vi "Index not Created Invalid path.vi"(8 "error in (no error)":errorcluster, 11 "Indexing Test Finder Test in":refnum<class "Indexing Test Finder Test.lvclass">) -> (0 "error out":errorcluster, 3 "Indexing Test Finder Test out":refnum<class "Indexing Test Finder Test.lvclass">)   [LabVIEW 2020, in "LUnit Tests.lvlib" / "Indexing Test Finder Test.lvclass"]
uses:
  Indexing Test Finder Test.lvclass
  Indexing Test Finder Test.lvclass/Indexing Test Finder Test.ctl
  source/Framework/Helper Classes/Test Finder/Test Finder.lvclass
  Test Finder/Finder Test.lvclass
  c59a45e6-8387-4d73-9fe8-839093b27eb6.vi
  <vilib>/Astemes/LUnit/Test Case.lvclass
  C:/Git/astemes-lunit/tests/Test Finder/Finder Test.lvclass
  C:/Program Files (x86)/National Instruments/LabVIEW 2020/vi.lib/Astemes/LUnit/Test Case.lvclass
  C:/Git/astemes-lunit/tests/Indexing Test Finder Test/Indexing Test Finder Test.lvclass
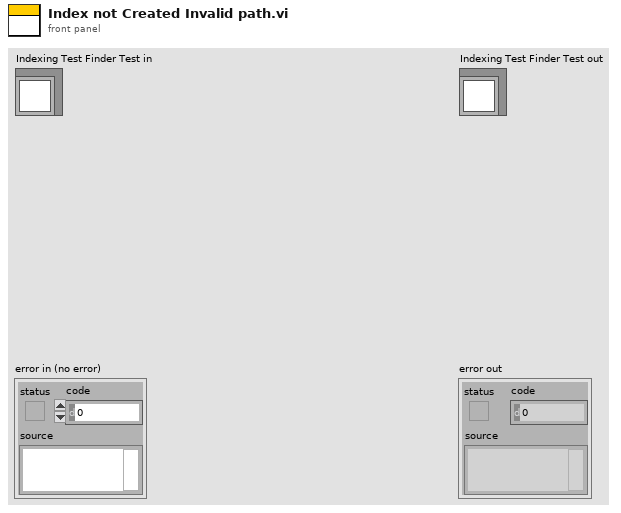
[diagram p1: front panel]
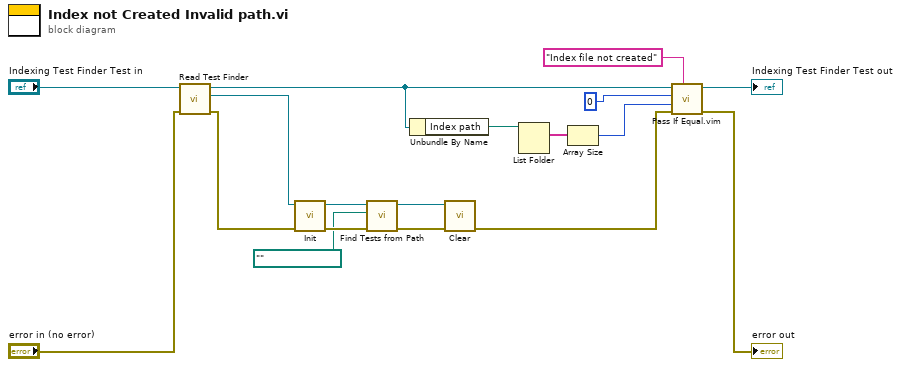
[diagram p0: block diagram]
diagram:
  n1 = call "Read Test Finder.vi"("error in (no error)"="error in (no error)", "Test Finder In"="Indexing Test Finder Test in") -> ("error out"=w12:errorcluster, "Test Finder.lvclass"=w13:refnum<class "Test Finder.lvclass">, "Test Finder Out"=w5:refnum<class "Indexing Test Finder Test.lvclass">)  [unwired: 7 in]
  n2 = call-dynamic "Init.vi"("error in (no error)"=w12, "Test Finder in"=w13) -> ("error out"=w16:errorcluster, "Test Finder out"=w17:refnum<class "Test Finder.lvclass">)  [unwired: 8 in]
  n3 = call-dynamic "Find Tests from Path.vi"("error in (no error)"=w16, "Project or Class Path"=path "", "Test Case Finder In"=w17) -> ("error out"=w14:errorcluster, "Test Case Finder Out"=w15:refnum<class "Test Finder.lvclass">)  [unwired: 7 in]
  n4 = Unbundle By Name(w5) -> ("Index path"=w9:path)
  n5 = call "Clear.vi"("error in (no error)"=w14, "Test Finder in"=w15) -> ("error out"=w10:errorcluster)  [unwired: 8 in, 1 out]
  n6 = List Folder(path=w9) -> (filenames=w8:string[])  [unwired: 3 in, 3 out]
  n7 = Array Size(array=w8) -> (size(s)=w4:i32)
  n8 = call "Pass If Equal.vim"("Description"="Index file not created", "error in (no error)"=w10, "Actual"=w4, "Expected"=0 ("size(s)"), "LUnit Test Case In"=w5) -> ("error out"=→"error out":errorcluster, "LUnit Test Case Out"=→"Indexing Test Finder Test out":refnum<class "Indexing Test Finder Test.lvclass">)  [unwired: 5 in]
